vi "Determine Optimal Setpoints.vi"(0 "Front Left":dbl, 2 "Front Right":dbl, 4 "Rear Left":dbl, 6 "Rear Right":dbl) -> (20 "Front Left Out":dbl, 21 "Front Right Out":dbl, 22 "Rear Left Out":dbl, 23 "Rear Right Out":dbl, 24 "Inv. Front Left Drive?":bool, 25 "Inv. Front Right Drive?":bool, 26 "Inv. Rear Left Drive?":bool, 27 "Inv. Rear Right Drive?":bool)   [LabVIEW 2012]
uses:
  Globals/Potentiometers.vi
panel:
  # "These are taken in as angles and output as absolute pot voltage."
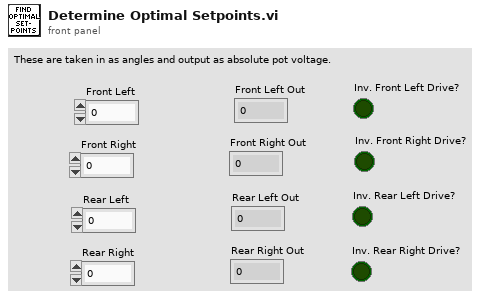
[diagram p1: front panel]
types:
  T1 = typedef "WPI_AnalogChannelDevRef.ctl" = cluster{"DevStatus":errorcluster, "Analog Module":T2, "Analog Channel":T3}
  T2 = typedef "FPGA_TypedefAnalogModule.ctl" = enum16{"Analog Module 1", "Analog Module 2"}
  T3 = typedef "FPGA_AIChannel.ctl" = enum8{"AI 1", "AI 2", "AI 3", "AI 4", "AI 5", "AI 6", "AI 7", "AI 8", "Invalid"}
  T4 = cluster{"Front Left":T1, "Front Right":T1, "Rear Left":T1, "Rear Right":T1, "Actuator":T1}
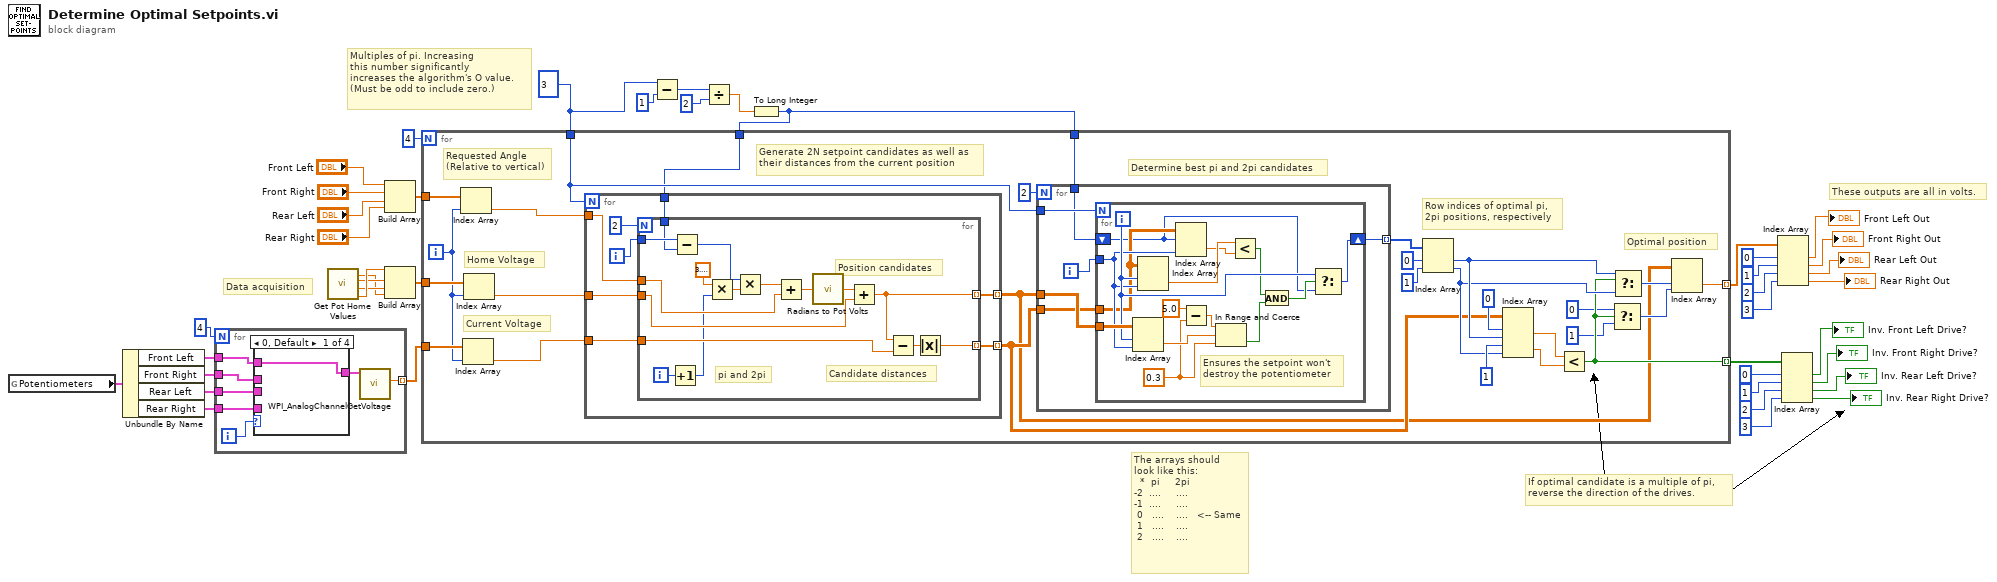
[diagram p0: block diagram]
diagram:
  w6 = 3
  # "If optimal candidate is a multiple of pi,\nreverse the direction of the drives."
  # "Data acquisition"
  # "Multiples of pi. Increasing\nthis number significantly\nincreases the algorithm's O value. \n(Must be odd to include zero.)"
  # "The arrays should \nlook like this:\n  *  pi     2pi\n-2  ....     ....\n-1  ....     ....\n 0   ....    ....   <-- Same\n 1   ....    ....\n 2   ....    ...."
  # "These outputs are all in volts."
  n1 = global read "Potentiometers.vi" "Potentiometers"() -> (w34:T4)
  n2 = Unbundle By Name(w34) -> ("Front Left"=w32:T1, "Front Right"=w31:T1, "Rear Left"=w30:T1, "Rear Right"=w29:T1)
  n3 = for {
    N: 4 -> [_]
    tunnel: w32 -> [w48]
    tunnel: w31 -> [w47]
    tunnel: w30 -> [w46]
    tunnel: w29 -> [w45]
    tunnel: [w43] -> w25 mode=indexing
    i -> [w49]
    n4 = case shown="0, Default" w49 {
      tunnel: w48 -> [w50 _ _ _]
      tunnel: w47 -> [_ w51 _ _]
      tunnel: w46 -> [_ _ w52 _]
      tunnel: w45 -> [_ _ _ w53]
      tunnel: [w50 w51 w52 w53] -> w44
      frame 0, Default {
      }
      frame 1 {
      }
      frame 2 {
      }
      frame 3 {
      }
    }
    n5 = call <vilib>:"WPI_AnalogChannelGetVoltage.vi"("AIDeviceRef"=w44) -> ("Voltage"=w43:dbl)  [unwired: 8 in, 2 out]
  }
  n6 = call "Get Pot Home Values.vi"() -> ("Front Left"=w38:dbl, "Rear Left"=w36:dbl, "Front Right"=w37:dbl, "Rear Right"=w35:dbl)  [unwired: 8 in]
  n7 = Build Array("Front Left", "Front Right", "Rear Left", "Rear Right") -> (w27:dbl[])
  n8 = Build Array(w38, w37, w36, w35) -> (w26:dbl[])
  n9 = Subtract(x=w6, y=1) -> (x-y=w4:i32)
  n10 = Divide(x=w4, y=2) -> (x/y=w2:dbl)
  n11 = To Long Integer(number=w2) -> (32bit integer=w1:i32)
  n12 = for {
    N: 4 -> [_]
    tunnel: w27 -> [w81]
    tunnel: w26 -> [w80]
    tunnel: w25 -> [w79]
    tunnel: [w63] -> w7 mode=indexing
    tunnel: [w66] -> w24 mode=indexing
    tunnel: w6 -> [w57]
    tunnel: w1 -> [w56]
    tunnel: w1 -> [w55]
    i -> [w78]
    # "Generate 2N setpoint candidates as well as\ntheir distances from the current position"
    # "Row indices of optimal pi,\n2pi positions, respectively"
    # "Optimal position"
    # "Determine best pi and 2pi candidates"
    # "Current Voltage"
    # "Home Voltage"
    # "Requested Angle\n(Relative to vertical)"
    n13 = Index Array(array=w81, index=w78) -> (element=w77:dbl)
    n14 = Index Array(array=w79, index=w78) -> (element=w74:dbl)
    n15 = Index Array(array=w80, index=w78) -> (element=w76:dbl)
    n16 = for {
      N: w57 -> [_]
      tunnel: w77 -> [w107]
      tunnel: w76 -> [w108]
      tunnel: [w106] -> w54 mode=indexing
      tunnel: w74 -> [w105]
      tunnel: [w104] -> w58 mode=indexing
      tunnel: w56 -> [w103]
      i -> [w109]
      n17 = for {
        N: 2 -> [_]
        tunnel: w109 -> [w124]
        tunnel: w108 -> [w117]
        tunnel: w107 -> [w118]
        tunnel: [w114] -> w106 mode=indexing
        tunnel: w105 -> [w115]
        tunnel: [w121] -> w104 mode=indexing
        tunnel: w103 -> [w113]
        i -> [w126]
        # "pi and 2pi"
        # "Candidate distances"
        # "Position candidates"
        n18 = Increment(x=w126) -> (x+1=w111:i32)
        n19 = Subtract(x=w124, y=w113) -> (x-y=w112:i32)
        n20 = Multiply(x=3.141592653589793, y=w111) -> (x*y=w123:dbl)
        n21 = Multiply(x=w112, y=w123) -> (x*y=w120:dbl)
        n22 = Add(x=w120, y=w118) -> (x+y=w119:dbl)
        n23 = call "Radians to Pot Volts.vi"("Angle In"=w119) -> ("Pot Delta Out"=w116:dbl)
        n24 = Add(x=w116, y=w117) -> (x+y=w114:dbl)
        n25 = Subtract(x=w114, y=w115) -> (x-y=w122:dbl)
        n26 = Absolute Value(x=w122) -> (abs(x)=w121:dbl)
      }
    }
    n27 = for {
      N: 2 -> [_]
      tunnel: w58 -> [w84]
      tunnel: w54 -> [w85]
      tunnel: [w86] -> w72 mode=indexing
      tunnel: w57 -> [w83]
      tunnel: w55 -> [w82]
      i -> [w87]
      n28 = for {
        N: w83 -> [_]
        tunnel: w87 -> [w96]
        tunnel: w84 -> [w95]
        tunnel: w85 -> [w102]
        shift-right: [w97] -> w86
        shift-left: w82 -> [w91]
        i -> [w98]
        w89 = 0.3 ("Safety volts")
        # "Ensures the setpoint won't\ndestroy the potentiometer"
        n29 = Index Array(array=w102, index (row)=w98, index (col)=w96) -> (element=w101:dbl)
        n30 = Index Array(array=w95, index (row)=w98, index (col)=w96) -> (element=w94:dbl)
        n31 = Index Array(array=w95, index (row)=w91, index (col)=w96) -> (element=w93:dbl)
        n32 = Subtract(x=5.0, y=w89) -> (x-y=w88:dbl)
        n33 = In Range and Coerce(upper limit=w88, x=w101, lower limit=w89) -> (In Range?=w100:bool)  [unwired: 1 out]
        n34 = Less?(x=w94, y=w93) -> (x < y?=w92:bool)
        n35 = And(x=w92, y=w100) -> (x .and. y?=w99:bool)
        n36 = Select(t=w98, s=w99, f=w91) -> (s? t:f=w97:i32)
      }
    }
    n37 = Index Array(array=w72, index #1=0 ("index"), index #2=1 ("index")) -> (element #1=w65:i32, element #2=w64:i32)
    n38 = Index Array(array=w58, index (row) #1=0 ("index (row)"), index (col) #1=w65, index (row) #2=1 ("index (row)"), index (col) #2=w64) -> (element #1=w68:dbl, element #2=w67:dbl)
    n39 = Less?(x=w68, y=w67) -> (x < y?=w63:bool)
    n40 = Select(t=0 ("index (row)"), s=w63, f=1 ("index (row)")) -> (s? t:f=w60:i32)
    n41 = Select(t=w65, s=w63, f=w64) -> (s? t:f=w59:i32)
    n42 = Index Array(array=w54, index (row)=w59, index (col)=w60) -> (element=w66:dbl)
  }
  n43 = Index Array(array=w24, index #1=0 ("index"), index #2=1 ("index"), index #3=2 ("index"), index #4=3 ("index")) -> (element #1=→"Front Left Out":dbl, element #2=→"Front Right Out":dbl, element #3=→"Rear Left Out":dbl, element #4=→"Rear Right Out":dbl)
  n44 = Index Array(array=w7, index #1=0 ("index"), index #2=1 ("index"), index #3=2 ("index"), index #4=3 ("index")) -> (element #1=→"Inv. Front Left Drive?":bool, element #2=→"Inv. Front Right Drive?":bool, element #3=→"Inv. Rear Left Drive?":bool, element #4=→"Inv. Rear Right Drive?":bool)
